vi "Add Scalar to Section.vi"(8 "error in":errorcluster, 10 "Scalar Data":T2, 11 "Item Ref in":T1 format="%.0x") -> (0 "error out":errorcluster, 3 "Item Ref out":T1 format="%.0x")   [LabVIEW 2019, in "Scripting API.lvlib"]
uses:
  Scripting API.lvlib
  <vilib>/NI VeriStand/Custom Device API/Custom Device Item Ref.ctl
  TypeDefs/Input Scalar Data.ctl
  Addon/Addon System Explorer/FPGA Addon System Explorer.lvlib
  <vilib>/NI VeriStand/Custom Device API/Custom Device API.lvlib
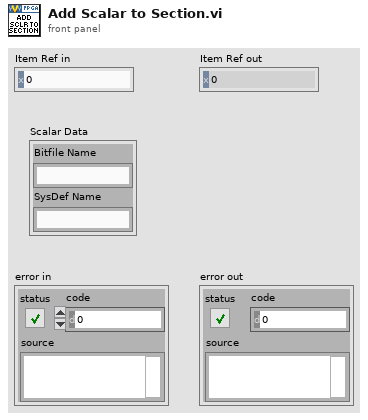
[diagram p1: front panel]
types:
  T1 = typedef "Custom Device API.lvlib/Custom Device Item Ref.ctl" = u64
  T2 = typedef "Scripting API.lvlib/Input Scalar Data.ctl" = cluster{"Bitfile Name":string, "SysDef Name":string}
  T3 = typedef "Scripting API.lvlib/Section Scalar Data.ctl" = cluster{"Scalar Section ref":T1, "Imported":bool, "Is Input":bool, "Register Information":T4}
  T4 = typedef "FPGA Addon Shared.lvlib/Register Information.ctl" = cluster{"Name":string, "Data Type":T5, "Default Value":variant, "Attributes":variant}
  T5 = typedef "FPGA Addon Shared.lvlib/FPGA Addon Data Type.ctl" = enum8{"<Null>", "I8", "I16", "I32", "I64", "U8", "U16", "U32", "U64", "SGL", "Boolean", "Analog PWM In Settings", "Analog PWM In", "Digital PWM In Settings", "Digital PWM In", "Digital PWM Out", "Sine Out", "FXP", "FXP+/-24.5", "FXP+/-16.5", "FXP+/-32.8", "FXP+/-64.32", "FXP+/-16.7", "FXP+/-20.5", "FXP+/-27.5", "FXP+/-32.16", "FXP+16.3", "FXP+18.3", "Digital Static In", "Digital Static Out", "Digital Static In Settings", "Digital WSS Out", "Quad Encoder Settings", "Quad Encoder In", "Group"}
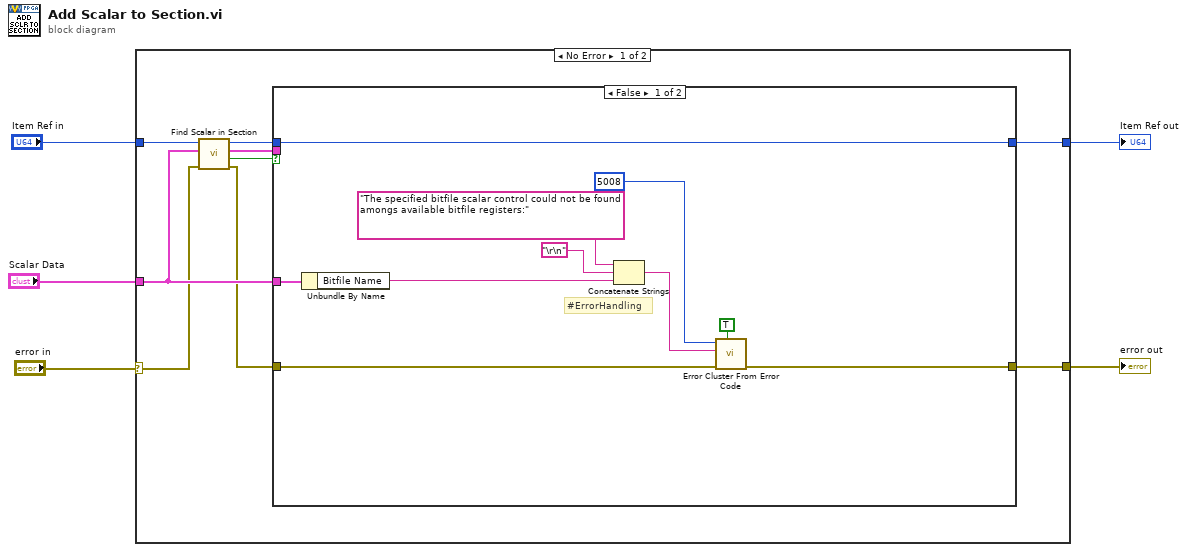
[diagram p0: block diagram]
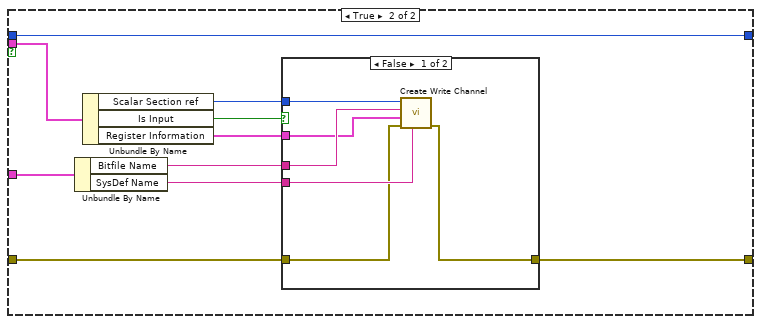
[diagram p2: hidden frame]
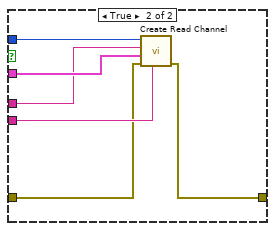
[diagram p3: hidden frame]
diagram:
  n1 = case shown="No Error" "error in" {
    selector: "error in" -> [w10 w48]
    tunnel: "Item Ref in" -> [w14 w47]
    tunnel: "Scalar Data" -> [w12 _]
    tunnel: [w7 w47] -> w4
    tunnel: [w6 w48] -> w5
    frame No Error {
      n2 = call "Find Scalar in Section.vi"("error in"=w10, "Scalar Data"=w12, "FPGA Addon refnum in"=w14) -> ("error out"=w9:errorcluster, "Found ?"=w11:bool, "Section Scalar Data"=w13:T3, "FPGA Addon refnum out"=w8:T1)  [unwired: 5 in]
      n3 = case shown="False" w11 {
        tunnel: w13 -> [_ w34]
        tunnel: w12 -> [w16 w30]
        tunnel: w9 -> [w18 w27]
        tunnel: w8 -> [w24 w26]
        tunnel: [w24 w26] -> w7
        tunnel: [w17 w25] -> w6
        frame False {
          # "#ErrorHandling"
          n4 = Unbundle By Name(w16) -> ("Bitfile Name"=w15:string)
          n5 = Concatenate Strings("The specified bitfile scalar control could not be found amongs available bitfile registers:" ("error message (\"\")"), "\r\n", w15) -> (w19:string)
          n6 = call <vilib>:"Error Cluster From Error Code.vi"("show call chain? (False)"=TRUE, "error in (no error)"=w18, "error message (\"\")"=w19, "error code (0)"=5008) -> ("error out"=w17:errorcluster)  [unwired: 5 in]
        }
        frame True {
          n7 = Unbundle By Name(w30) -> ("Bitfile Name"=w29:string, "SysDef Name"=w28:string)
          n8 = Unbundle By Name(w34) -> ("Scalar Section ref"=w32:T1, "Is Input"=w33:bool, "Register Information"=w31:T4)
          n9 = case shown="False" w33 {
            tunnel: w32 -> [w40 w46]
            tunnel: w31 -> [w38 w45]
            tunnel: w29 -> [w39 w44]
            tunnel: w28 -> [w37 w43]
            tunnel: w27 -> [w36 w42]
            tunnel: [w35 w41] -> w25
            frame False {
              n10 = call "Create Write Channel.vi"("Name"=w37, "error in (no error)"=w36, "Cluster"=w38, "Bitfile Name"=w39, "Item Ref in"=w40) -> ("error out"=w35:errorcluster)  [unwired: 6 in]
            }
            frame True {
              n11 = call "Create Read Channel.vi"("Name"=w43, "error in (no error)"=w42, "Channel"=w45, "Bitfile Name"=w44, "Item Ref in"=w46) -> ("error out"=w41:errorcluster)  [unwired: 6 in]
            }
          }
        }
      }
    }
    frame Error {
    }
  }
  "error out" <- w5
  "Item Ref out" <- w4
